vi "Read Configuration.vi"(8 "file path (trajectorymat)":path=path "c:/ni-rt/startup/trajectorymat.csv", 9 "file path (matrixmat)":path=path "c:/ni-rt/startup/matrixmat_tuned_QR_7.csv", 10 "XML File Path conf":path=path "c:/ni-rt/startup/configuration.xml", 11 "Error In":errorcluster) -> (0 "values loded in xml files":T2, 1 "configuration":T1={"Accelerometer Bias"={"X (m/s)"=0.0, "Y (m/s)"=0.0, "Z (m/s)"=0.0}, "Gyroscope Bias"={"X (m/s)"=0.0, "Y (m/s)"=0.0, "Z (m/s)"=0.0}, "Steering Motor Gear Ratio"=111.0, "Steering Pully Gear Ratio"=1.0, "Steering Encoder CPR"=500.0, "Steering Motor Max RPM"=4000.0, "Wheelbase (m)"=1.12, "Fork Angle (rad)"=1.3, "Balancing Controller"={"Kp (/s)"=1.3, "Kd (1)"=3.0}, "Max Allowed Steering Angle (rad)"=0.7, "Task Periods"={"Emergency Stop (us)"=10000, "IMU (us)"=10000, "Steering Motor Encoder (us)"=10000, "State Estimator (us)"=10000, "Balancing Controller (us)"=10000, "GNSS (us)"=10000, "Logging (us)"=50000, "Drive Motor (us)"=100000, "Visualization (us)"=100000}, "Drive Motor Gear Ratio"=250.0, "lr"=0.4964, "lf"=0.5986, "lambda"=1.2217, "k1"=0.004472, "k2"=0.09678, "e1_max"=11.331, "Ad_t"=0.95971, "Bd_t"=0.01, "C_t"=2.20588, "D_t"=0.0, "Wheel radius"=0.311}, 2 "value":T3, 3 "error out":errorcluster, 4 "Trajectory":T3, 5 "Init trajectory (2)":dbl[][](array[numeric]), 6 "Matrix Matlab":T3)   [LabVIEW 2021]
uses:
  <vilib>/Analysis/Matrix/Datatypes/RealMatrix.ctl
  Configuration.ctl
  <vilib>/Utility/xml.llb/Read From XML File(string).vi
  <vilib>/Analysis/Matrix/Numeric/Conversions/Matrix To Array - RM.vi
  <vilib>/Utility/file.llb/Read Delimited Spreadsheet (DBL).vi
  <vilib>/Analysis/Matrix/NI_Matrix.lvlib
panel:
  in  "delimiter (,) 2":string=","
  in  "error in (no error) 2":errorcluster
  in  "delimiter (,)":string=","
  in  "error in (no error)":errorcluster
  in  "init trajectory":dbl[][](array[numeric])
  in  "XML File Path traj":path=path "c:/ni-rt/startup/trajectorylab.xml"
  in  "Init Matrix":T3
  in  "XML File Path matr":path=path "c:/ni-rt/startup/matrixlab.xml"
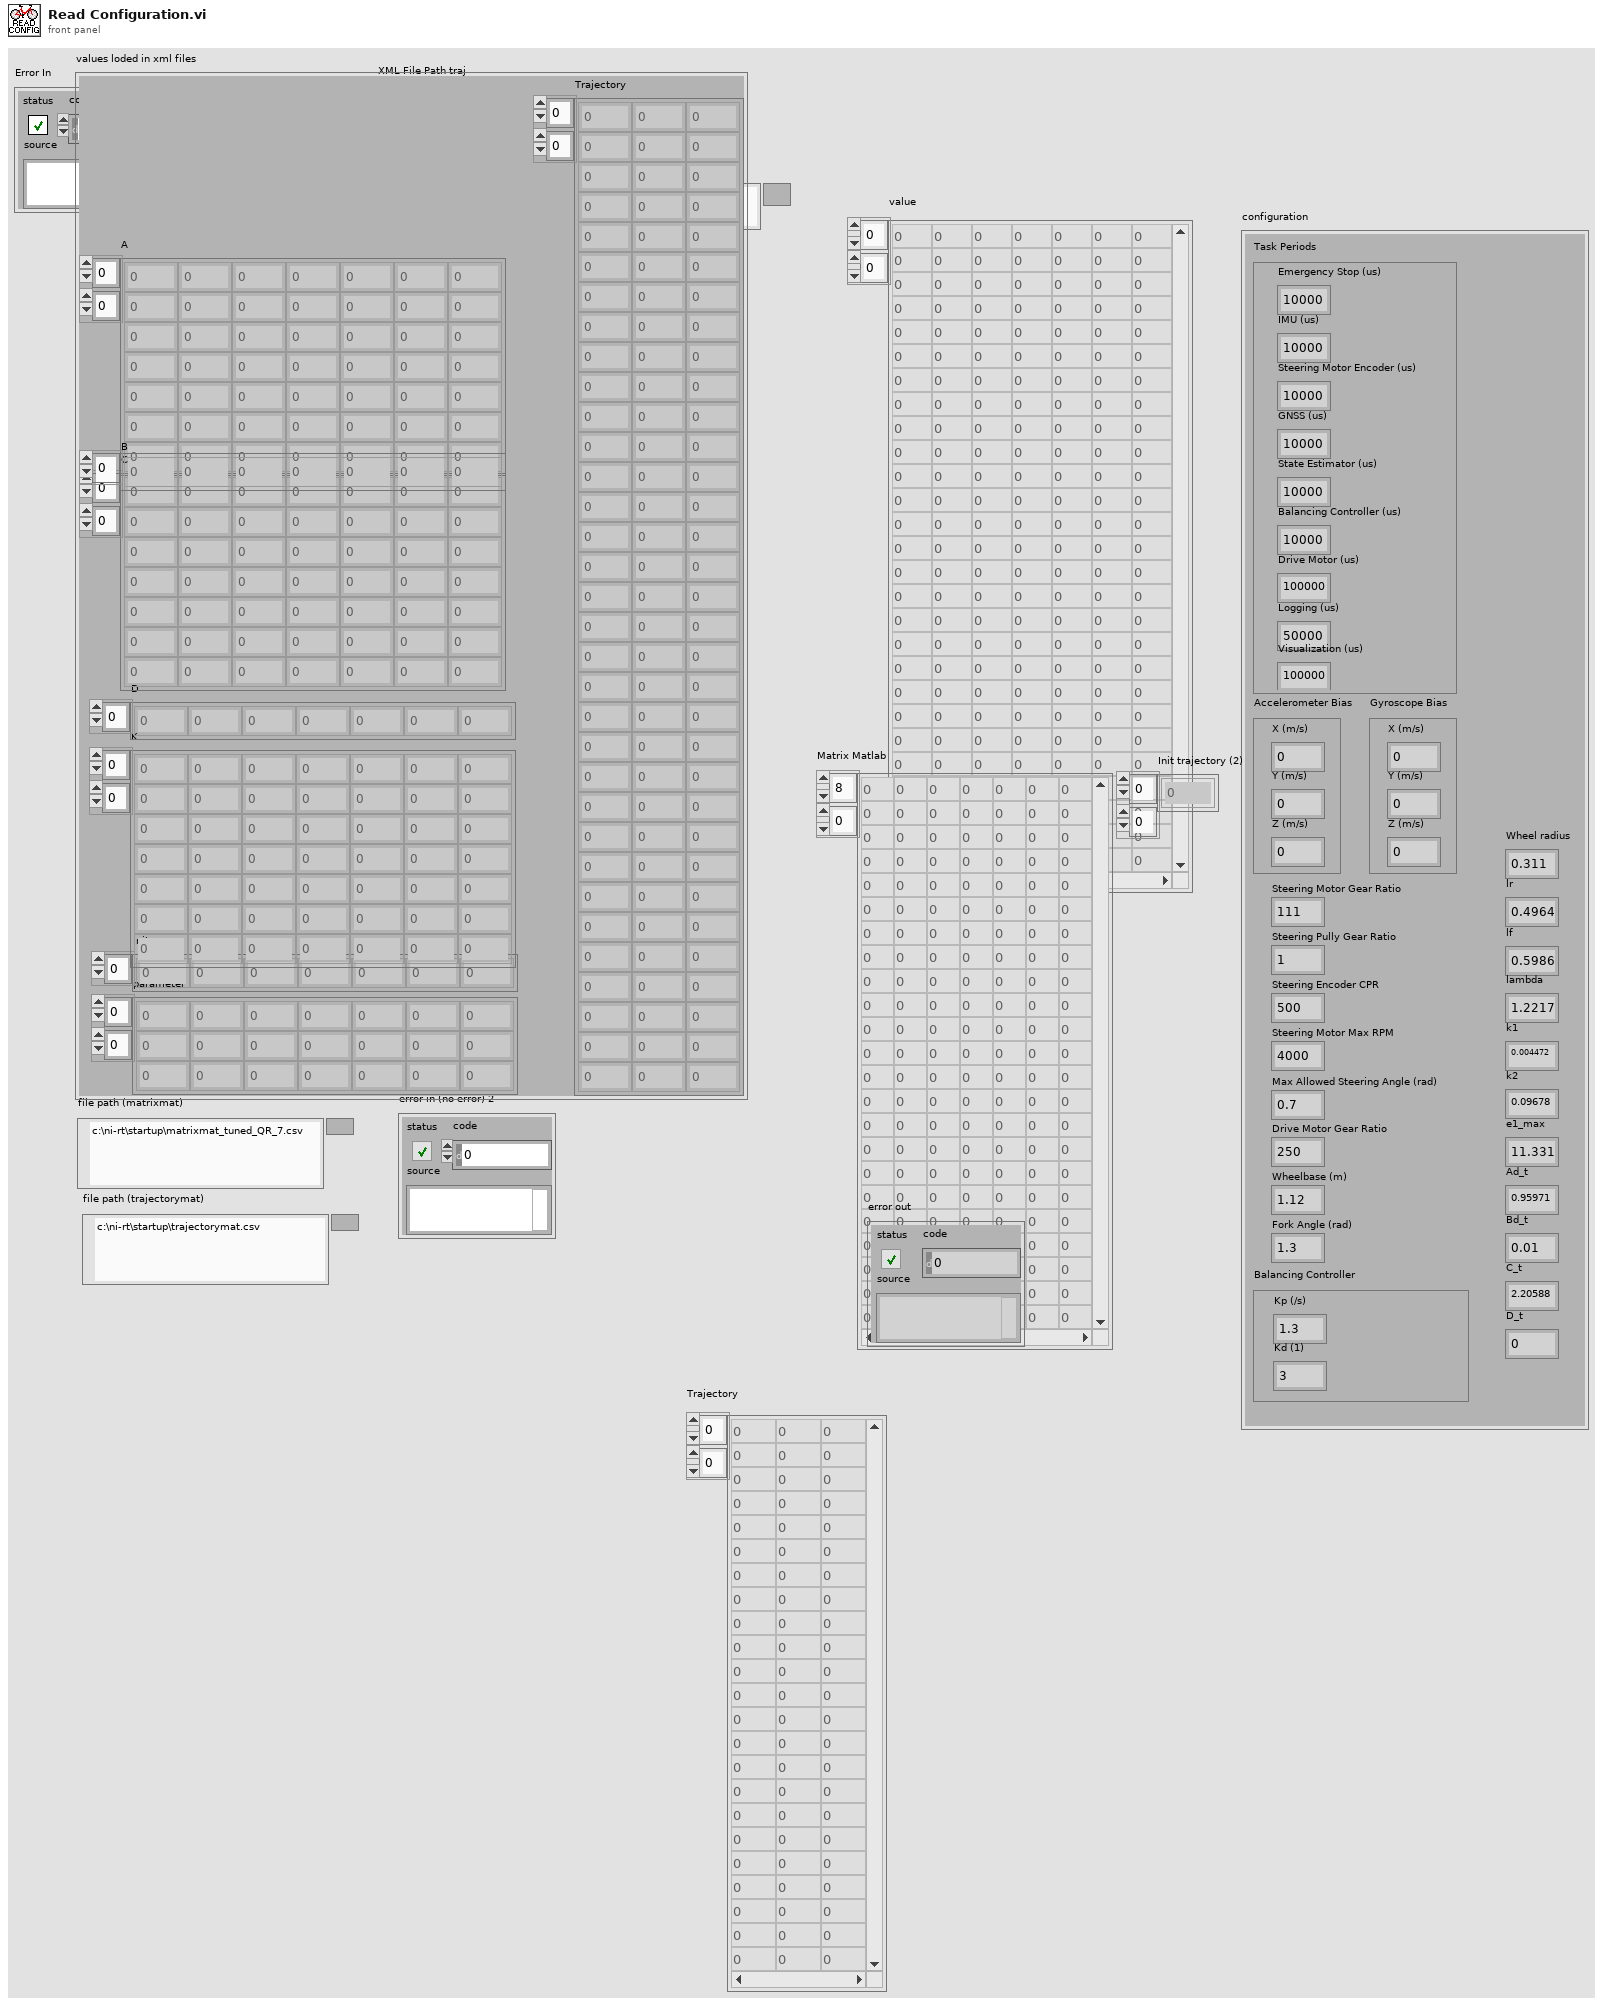
[diagram p1: front panel]
types:
  T1 = typedef "Configuration.ctl" = cluster{"Accelerometer Bias":cluster{"X (m/s)":dbl, "Y (m/s)":dbl, "Z (m/s)":dbl}, "Gyroscope Bias":cluster{"X (m/s)":dbl, "Y (m/s)":dbl, "Z (m/s)":dbl}, "Steering Motor Gear Ratio":dbl, "Steering Pully Gear Ratio":dbl, "Steering Encoder CPR":dbl, "Steering Motor Max RPM":dbl, "Wheelbase (m)":dbl, "Fork Angle (rad)":dbl, "Balancing Controller":cluster{"Kp (/s)":dbl, "Kd (1)":dbl}, "Max Allowed Steering Angle (rad)":dbl, "Task Periods":cluster{"Emergency Stop (us)":i64, "IMU (us)":i64, "Steering Motor Encoder (us)":i64, "State Estimator (us)":i64, "Balancing Controller (us)":i64, "GNSS (us)":i64, "Logging (us)":i64, "Drive Motor (us)":i64, "Visualization (us)":i64}, "Drive Motor Gear Ratio":dbl, "lr":dbl, "lf":dbl, "lambda":dbl, "k1":dbl, "k2":dbl, "e1_max":dbl, "Ad_t":dbl, "Bd_t":dbl, "C_t":dbl, "D_t":dbl, "Wheel radius":dbl}
  T2 = cluster{"B":dbl[], "A":dbl[][], "C":dbl[][], "D":dbl[], "K":dbl[][], "Trajectory":dbl[][], "Init":dbl[], "parameter":dbl[][]}
  T3 = typedef "NI_Matrix.lvlib/RealMatrix.ctl" = dbl[][]
  T4 = cluster{"[0]":dbl, "[1]":dbl, "[2]":dbl, "[3]":dbl, "[4]":dbl, "[5]":dbl, "[6]":dbl, "[7]":dbl, "[8]":dbl, "[9]":dbl, "[10]":dbl, "[11]":dbl, "[12]":dbl, "[13]":dbl, "[14]":dbl, "[15]":dbl, "[16]":dbl, "[17]":dbl, "[18]":dbl, "[19]":dbl, "[20]":dbl}
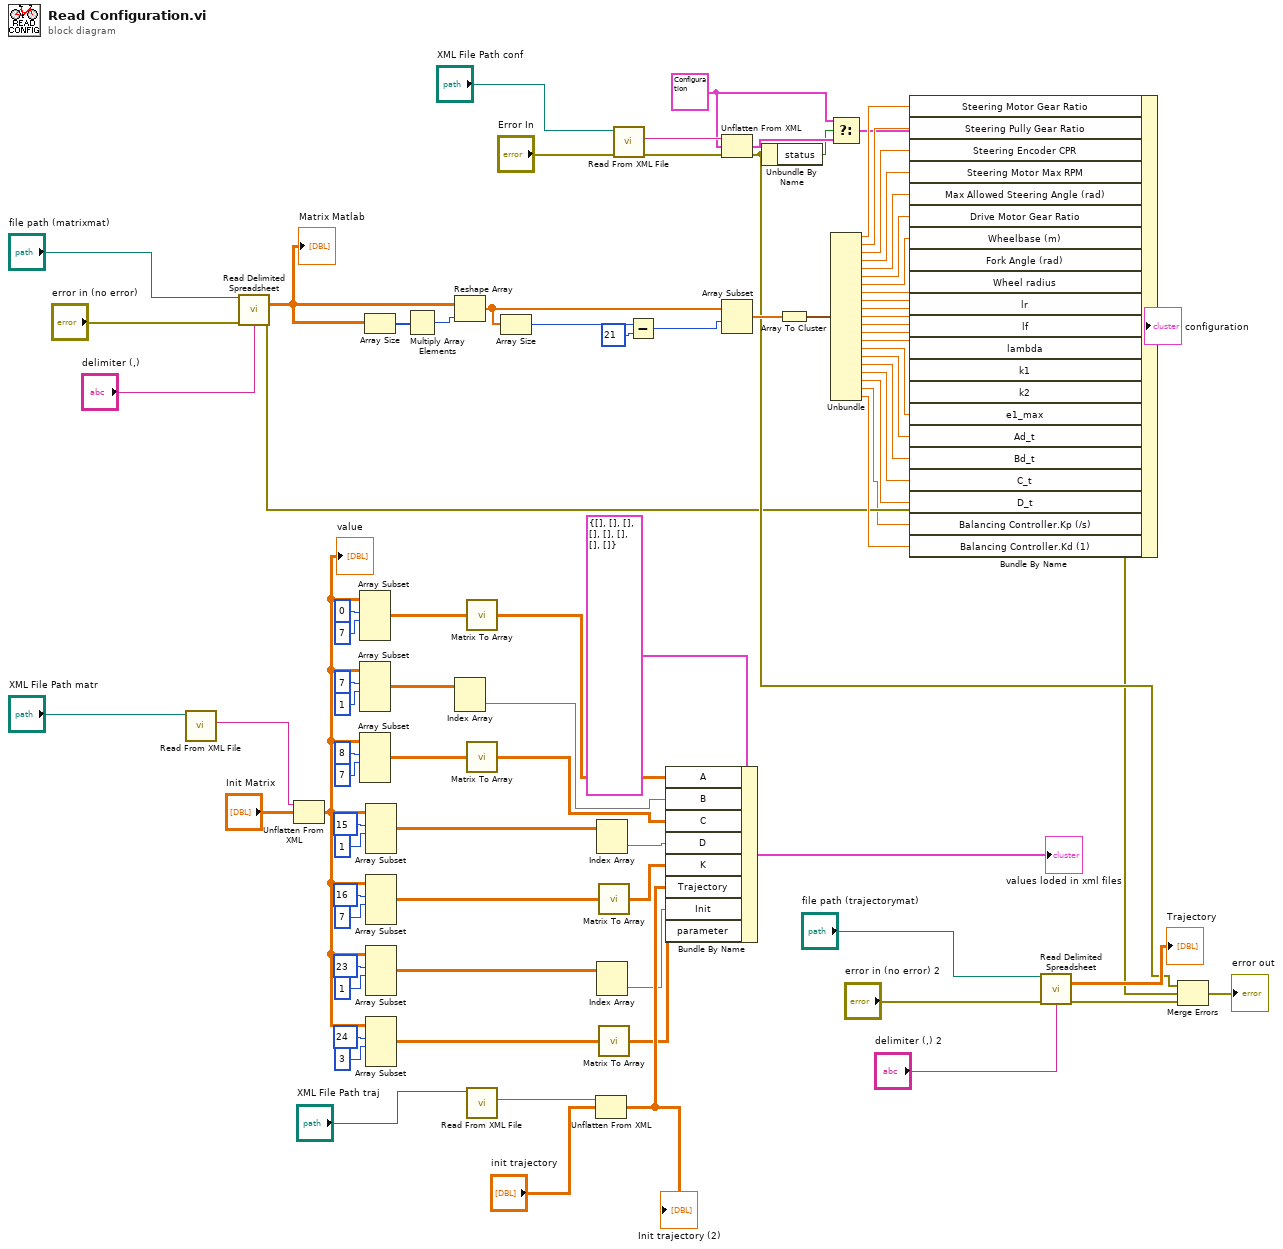
[diagram p0: block diagram]
diagram:
  w8 = T1 {"Accelerometer Bias"={"X (m/s)"=0.0, "Y (m/s)"=0.0, "Z (m/s)"=0.0}, "Gyroscope Bias"={"X (m/s)"=0.0, "Y (m/s)"=0.0, "Z (m/s)"=0.0}, "Steering Motor Gear Ratio"=611.0, "Steering Pully Gear Ratio"=1.0, "Steering Encoder CPR"=500.0, "Steering Motor Max RPM"=4000.0, "Wheelbase (m)"=1.12, "Fork Angle (rad)"=1.3, "Balancing Controller"={"Kp (/s)"=0.0, "Kd (1)"=0.0}, "Max Allowed Steering Angle (rad)"=0.7, "Task Periods"={"Emergency Stop (us)"=0, "IMU (us)"=0, "Steering Motor Encoder (us)"=0, "State Estimator (us)"=0, "Balancing Controller (us)"=0, "GNSS (us)"=0, "Logging (us)"=0, "Drive Motor (us)"=0, "Visualization (us)"=50000}, "Drive Motor Gear Ratio"=0.7, "lr"=0.0, "lf"=0.0, "lambda"=0.0, "k1"=0.0, "k2"=0.0, "e1_max"=0.0, "Ad_t"=0.0, "Bd_t"=0.0, "C_t"=0.0, "D_t"=0.0, "Wheel radius"=0.311} ("Configuration")
  n1 = call-poly <vilib>:"Read From XML File.vi"("XML File Path"="XML File Path matr") -> ("XML Elements"=w82:string)  [unwired: 8 in, 2 out]
  n2 = call-poly <vilib>:"Read Delimited Spreadsheet.vi"("file path (dialog if empty)"="file path (matrixmat)", "error in (no error)"="error in (no error)", "delimiter (\\t)"="delimiter (,)") -> ("all rows"=w32:dbl[][], "error out"=w3:errorcluster)  [unwired: 7 in, 4 out]
  "Matrix Matlab" <- w32
  n3 = Unflatten From XML(xml string=w82, type="Init Matrix") -> (value=w42:T3)  [unwired: 1 in, 1 out]
  "value" <- w42
  n4 = Array Subset(array=w42, index (row)=0, length (row)=7) -> (w78:T3)  [unwired: 2 in]
  n5 = Array Subset(array=w42, index (row)=7, length (row)=1) -> (w66:T3)  [unwired: 2 in]
  n6 = Array Subset(array=w42, index (row)=8, length (row)=7) -> (w72:T3)  [unwired: 2 in]
  n7 = Array Size(array=w32) -> (size(s)=w37:i32[])
  n8 = Array Subset(array=w42, index (row)=15, length (row)=1) -> (w62:T3)  [unwired: 2 in]
  n9 = Array Subset(array=w42, index (row)=16, length (row)=7) -> (w68:T3)  [unwired: 2 in]
  n10 = Array Subset(array=w42, index (row)=23, length (row)=1) -> (w53:T3)  [unwired: 2 in]
  n11 = Array Subset(array=w42, index (row)=24, length (row)=3) -> (w41:T3)  [unwired: 2 in]
  n12 = Multiply Array Elements(1:w37) -> (0:w36:i32)
  n13 = Reshape Array(w32, w36) -> (w31:dbl[])
  n14 = Index Array(array=w66) -> (element=w63:dbl[])  [unwired: 2 in]
  n15 = call-poly <vilib>:"Matrix To Array.vi"("Real Matrix"=w78) -> ("Real 2D Array"=w77:dbl[][])
  n16 = call-poly <vilib>:"Matrix To Array.vi"("Real Matrix"=w72) -> ("Real 2D Array"=w71:dbl[][])
  n17 = call-poly <vilib>:"Read From XML File.vi"("XML File Path"="XML File Path traj") -> ("XML Elements"=w59:string)  [unwired: 8 in, 2 out]
  n18 = Array Size(array=w31) -> (size(s)=w34:i32)
  n19 = Unflatten From XML(xml string=w59, type="init trajectory") -> (value=w56:dbl[][])  [unwired: 1 in, 1 out]
  "Init trajectory (2)" <- w56
  n20 = Index Array(array=w62) -> (element=w61:dbl[])  [unwired: 2 in]
  n21 = Index Array(array=w53) -> (element=w52:dbl[])  [unwired: 2 in]
  n22 = call-poly <vilib>:"Matrix To Array.vi"("Real Matrix"=w68) -> ("Real 2D Array"=w67:dbl[][])
  n23 = call-poly <vilib>:"Matrix To Array.vi"("Real Matrix"=w41) -> ("Real 2D Array"=w40:dbl[][])
  n24 = call-poly <vilib>:"Read From XML File.vi"("error in (no error)"="Error In", "XML File Path"="XML File Path conf") -> ("error out"=w88:errorcluster, "XML Elements"=w87:string)  [unwired: 7 in, 1 out]
  n25 = Subtract(x=w34, y=21 ("length")) -> (x-y=w33:i32)
  n26 = Bundle By Name(cluster=T2 {"B"=[], "A"=[], "C"=[], "D"=[], "K"=[], "Trajectory"=[], "Init"=[], "parameter"=[]} ("Matrix 2"), "A"=w77, "B"=w63, "C"=w71, "D"=w61, "K"=w67, "Trajectory"=w56, "Init"=w52, "parameter"=w40) -> (→"values loded in xml files":T2)
  n27 = Unflatten From XML(xml string=w87, type=w8, error in (no error)=w88) -> (value=w84:T1, error out=w4:errorcluster)
  n28 = Array Subset(array=w31, index=w33) -> (w30:dbl[])  [unwired: 1 in]
  n29 = Unbundle By Name(w4) -> ("status"=w81:bool)
  n30 = Array To Cluster(array=w30) -> (cluster=w29:T4)
  n31 = Select(t=w8, s=w81, f=w84) -> (s? t:f=w7:T1)
  n32 = Unbundle(w29) -> ("[0]"=w28:dbl, "[1]"=w27:dbl, "[2]"=w26:dbl, "[3]"=w25:dbl, "[4]"=w24:dbl, "[5]"=w23:dbl, "[6]"=w22:dbl, "[7]"=w21:dbl, "[8]"=w20:dbl, "[9]"=w19:dbl, "[10]"=w18:dbl, "[11]"=w17:dbl, "[12]"=w16:dbl, "[13]"=w15:dbl, "[14]"=w14:dbl, "[15]"=w13:dbl, "[16]"=w12:dbl, "[17]"=w11:dbl, "[18]"=w10:dbl, "[19]"=w1:dbl, "[20]"=w9:dbl)
  n33 = Bundle By Name(cluster=w7, "Steering Motor Gear Ratio"=w28, "Steering Pully Gear Ratio"=w27, "Steering Encoder CPR"=w26, "Steering Motor Max RPM"=w25, "Max Allowed Steering Angle (rad)"=w24, "Drive Motor Gear Ratio"=w23, "Wheelbase (m)"=w22, "Fork Angle (rad)"=w21, "Wheel radius"=w20, "lr"=w19, "lf"=w18, "lambda"=w17, "k1"=w16, "k2"=w15, "e1_max"=w14, "Ad_t"=w13, "Bd_t"=w12, "C_t"=w11, "D_t"=w10, "Balancing Controller.Kp (/s)"=w1, "Balancing Controller.Kd (1)"=w9) -> (→"configuration":T1)
  n34 = call-poly <vilib>:"Read Delimited Spreadsheet.vi"("file path (dialog if empty)"="file path (trajectorymat)", "error in (no error)"="error in (no error) 2", "delimiter (\\t)"="delimiter (,) 2") -> ("all rows"=→"Trajectory":dbl[][], "error out"=w2:errorcluster)  [unwired: 7 in, 4 out]
  n35 = Merge Errors(w4, w3, w2) -> (→"error out":errorcluster)
